vi "Test_Result.vi"(9 "Load Time":i32, 10 "Preload Time":i32, 11 "Tripped Time":i32[](array[numeric])) -> (2 "Pass/Fail?":bool)   [LabVIEW 2015]
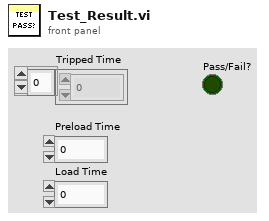
[diagram p1: front panel]
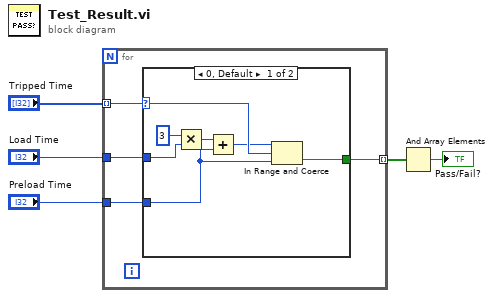
[diagram p0: block diagram]
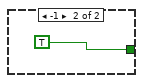
[diagram p2: hidden frame]
diagram:
  n1 = for {
    tunnel: "Preload Time" -> [w8]
    tunnel: "Load Time" -> [w9]
    tunnel: "Tripped Time" -> [w6] mode=indexing
    tunnel: [w7] -> w2 mode=indexing
    n2 = case shown="0, Default" w6 {
      selector: w6 -> [w12 _]
      tunnel: w9 -> [w14 _]
      tunnel: w8 -> [w10 _]
      tunnel: [w13 TRUE] -> w7
      frame 0, Default {
        n3 = Multiply(x=3, y=w14) -> (x*y=w16:i32)
        n4 = Add(x=w16, y=w10) -> (x+y=w11:i32)
        n5 = In Range and Coerce(upper limit=w11, x=w12, lower limit=w10) -> (In Range?=w13:bool)  [unwired: 1 out]
      }
      frame -1 {
      }
    }
  }
  n6 = And Array Elements(Boolean array=w2) -> (logical AND=→"Pass/Fail?":bool)
